vi "robot.vi"() -> ()   [LabVIEW 2016]
uses:
  <vilib>/Instr/_visa.llb/VISA Configure Serial Port (Instr).vi
panel:
  in  "?":i32
  out "Score":i32
  out "Objects (pixel) (Object Tracking 1)":T1(array[cluster])
  out "object found ?":bool
  in  "Stop (F)":bool
  out "?":T2(plugin-control)
  in  "VISA resource name 2":refnum<visa-resource-name>
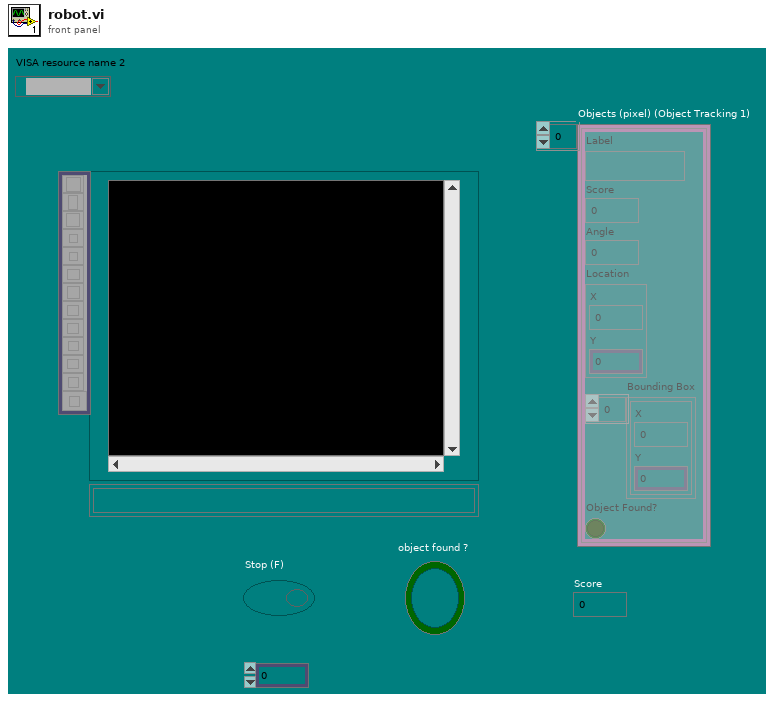
[diagram p1: front panel]
types:
  T1 = cluster{"Label":string, "Score":i32, "Angle":dbl, "Location":cluster{"X":dbl, "Y":dbl}, "Bounding Box":cluster{"X":dbl, "Y":dbl}[], "Object Found?":bool}[]
  T2 = typedef "IMAQ Image.ctl" = refnum<image>
  T3 = cluster{"Objects (pixel) (Object Tracking 1)[0]":cluster{"Label":string, "Score":i32, "Angle":dbl, "Location":cluster{"X":dbl, "Y":dbl}, "Bounding Box":cluster{"X":dbl, "Y":dbl}[], "Object Found?":bool}, "Objects (pixel) (Object Tracking 1)[1]":cluster{"Label":string, "Score":i32, "Angle":dbl, "Location":cluster{"X":dbl, "Y":dbl}, "Bounding Box":cluster{"X":dbl, "Y":dbl}[], "Object Found?":bool}, "Objects (pixel) (Object Tracking 1)[2]":cluster{"Label":string, "Score":i32, "Angle":dbl, "Location":cluster{"X":dbl, "Y":dbl}, "Bounding Box":cluster{"X":dbl, "Y":dbl}[], "Object Found?":bool}, "Objects (pixel) (Object Tracking 1)[3]":cluster{"Label":string, "Score":i32, "Angle":dbl, "Location":cluster{"X":dbl, "Y":dbl}, "Bounding Box":cluster{"X":dbl, "Y":dbl}[], "Object Found?":bool}, "Objects (pixel) (Object Tracking 1)[4]":cluster{"Label":string, "Score":i32, "Angle":dbl, "Location":cluster{"X":dbl, "Y":dbl}, "Bounding Box":cluster{"X":dbl, "Y":dbl}[], "Object Found?":bool}, "Objects (pixel) (Object Tracking 1)[5]":cluster{"Label":string, "Score":i32, "Angle":dbl, "Location":cluster{"X":dbl, "Y":dbl}, "Bounding Box":cluster{"X":dbl, "Y":dbl}[], "Object Found?":bool}, "Objects (pixel) (Object Tracking 1)[6]":cluster{"Label":string, "Score":i32, "Angle":dbl, "Location":cluster{"X":dbl, "Y":dbl}, "Bounding Box":cluster{"X":dbl, "Y":dbl}[], "Object Found?":bool}, "Objects (pixel) (Object Tracking 1)[7]":cluster{"Label":string, "Score":i32, "Angle":dbl, "Location":cluster{"X":dbl, "Y":dbl}, "Bounding Box":cluster{"X":dbl, "Y":dbl}[], "Object Found?":bool}, "Objects (pixel) (Object Tracking 1)[8]":cluster{"Label":string, "Score":i32, "Angle":dbl, "Location":cluster{"X":dbl, "Y":dbl}, "Bounding Box":cluster{"X":dbl, "Y":dbl}[], "Object Found?":bool}}
  T4 = cluster{"Label":string, "Score":i32, "Angle":dbl, "Location":cluster{"X":dbl, "Y":dbl}, "Bounding Box":cluster{"X":dbl, "Y":dbl}[], "Object Found?":bool}
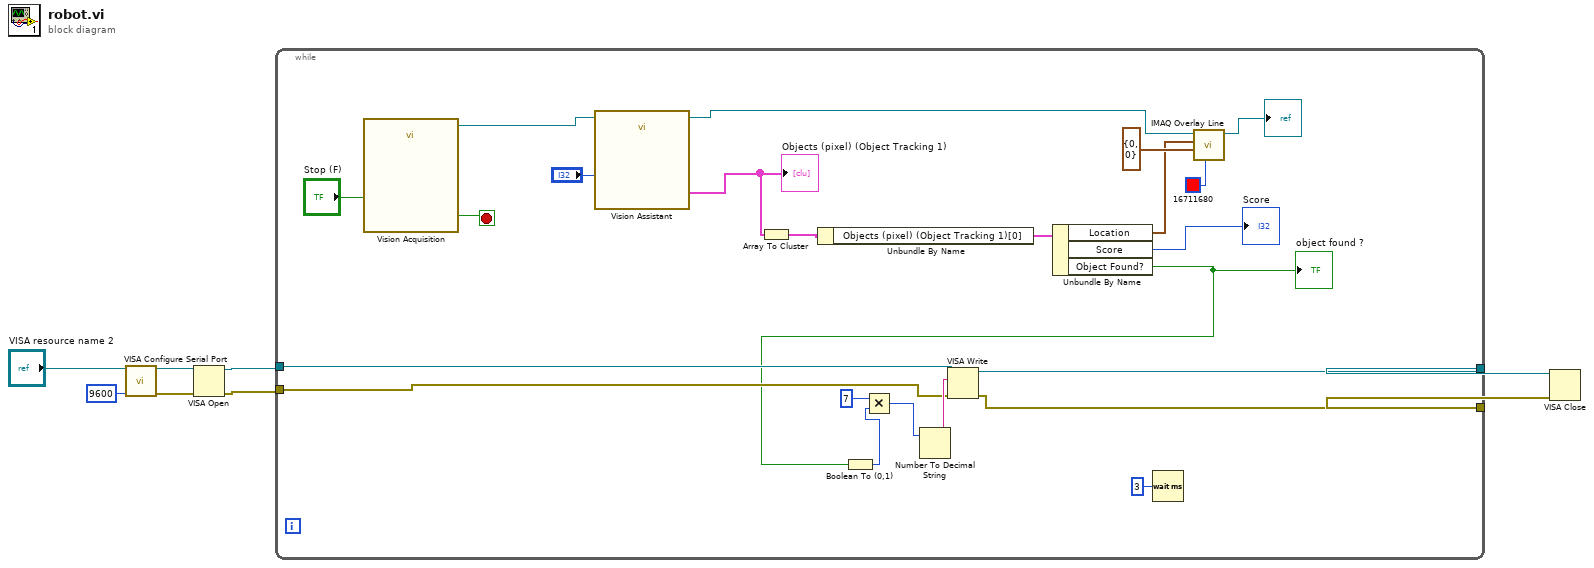
[diagram p0: block diagram]
diagram:
  n1 = call-poly "VISA Configure Serial Port"("VISA resource name"="VISA resource name 2", "baud rate (9600)"=u32 9600) -> ("VISA resource name out"=w5:refnum<visa-resource-name>, "error out"=w2:errorcluster)  [unwired: 12 in]
  n2 = VISA Open(error in (no error)=w2, VISA resource name=w5) -> (VISA resource name=w4:refnum<visa-resource-name>, error out=w3:errorcluster)  [unwired: 3 in]
  n3 = while {
    tunnel: [w26] -> w8
    tunnel: [w25] -> w7
    tunnel: w4 -> [w28]
    tunnel: w3 -> [w27]
    stop <- w11 stop-if-true
    n4 = call "Vision Acquisition"("Stop (F)"="Stop (F)") -> ("Image Out"=w18:T2, "Stopped"=w11:bool)  [unwired: 24 in, 1 out]
    n5 = call "Vision Assistant"("Image In"=w18, "Minimum Score (Object Tracking 1)"="?") -> ("Image Out"=w19:T2, "Objects (pixel) (Object Tracking 1)"=w14:T1)  [unwired: 23 in, 1 out]
    "Objects (pixel) (Object Tracking 1)" <- w14
    n6 = Array To Cluster(array=w14) -> (cluster=w17:T3)
    n7 = Unbundle By Name(w17) -> ("Objects (pixel) (Object Tracking 1)[0]"=w15:T4)
    n8 = Unbundle By Name(w15) -> ("Location"=w16:cluster{"X":dbl, "Y":dbl}, "Score"=→"Score":i32, "Object Found?"=w10:bool)
    "object found ?" <- w10
    n9 = Boolean To (0,1)(Boolean=w10) -> (0, 1=w30:i16)
    n10 = Multiply(x=i16 7, y=w30) -> (x*y=w31:i16)
    n11 = Number To Decimal String(number=w31) -> (decimal integer string=w29:string)  [unwired: 1 in]
    n12 = VISA Write(VISA resource name=w28, write buffer=w29, error in (no error)=w27) -> (VISA resource name out=w26:refnum<visa-resource-name>, error out=w25:errorcluster)  [unwired: 1 out]
    n13 = Wait (ms)(milliseconds to wait=u32 3) -> ()  [unwired: 1 out]
    n14 = call "IMAQ Overlay Line"("Color"=u32 16711680, "End Point"=cluster{"X":i32, "Y":i32} {"X"=0, "Y"=0}, "Start Point"=w16, "Image"=w19) -> ("Image Out"=→"?":T2)  [unwired: 6 in, 1 out]
  }
  n15 = VISA Close(VISA resource name=w8, error in (no error)=w7) -> ()  [unwired: 1 out]
